vi "SetI.vi"(8 "error in (no error)":errorcluster, 10 "i":i32, 11 "reference in":refnum<class "GOOP4_Sub.lvclass">) -> (0 "error out":errorcluster, 3 "reference in":refnum<class "GOOP4_Sub.lvclass">)   [LabVIEW 2019, in "GOOP4_Sub.lvclass"]
uses:
  GOOP4_Sub.lvclass
  C:/Users/Tiba/Desktop/GOOP4_CreateObjects_Open_GDS/GOOP4_Base_class/GOOP4_Base.lvclass
  GOOP4_Base_class/GOOP4_Base.lvclass
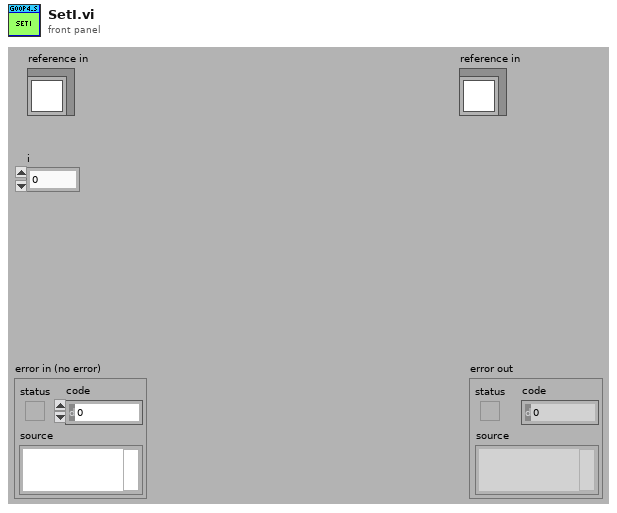
[diagram p1: front panel]
types:
  T1 = typedef "GOOP4_Base.lvclass/ObjectAttributes.ctl" = cluster{"i":i32}
  T2 = typedef "GOOP4_Sub.lvclass/ObjectAttributes.ctl" = cluster{"Str":string, "Boolean":bool}
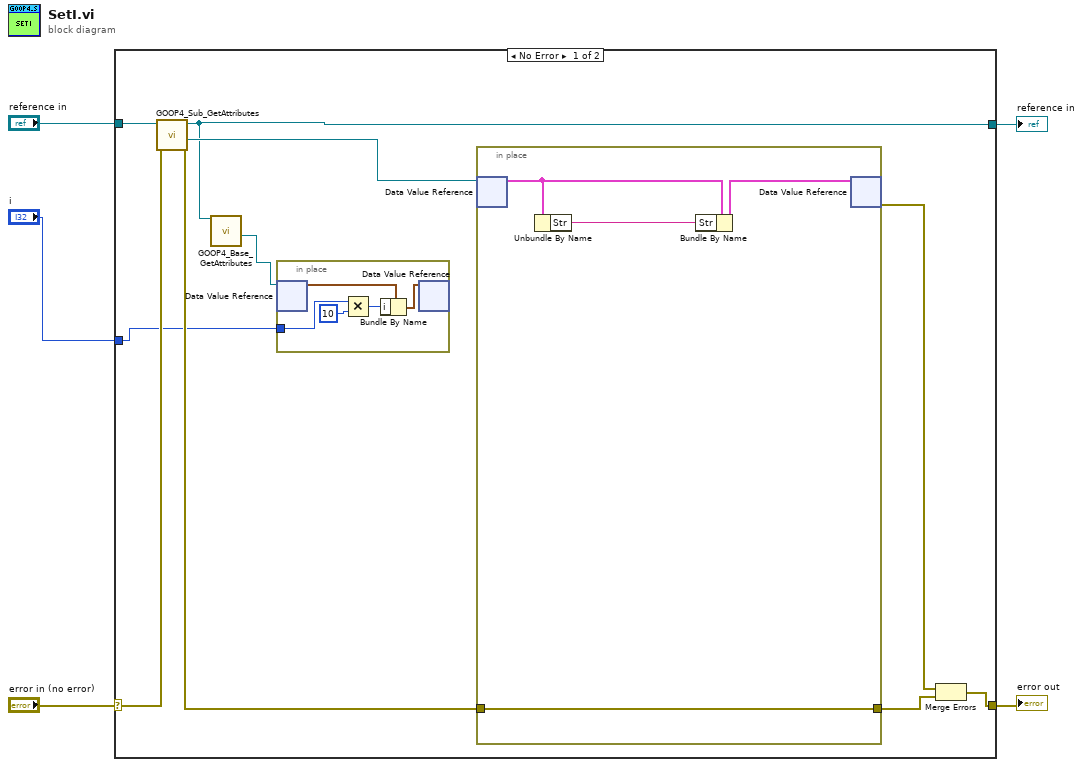
[diagram p0: block diagram]
diagram:
  n1 = case shown="No Error" "error in (no error)" {
    selector: "error in (no error)" -> [w14 w26]
    tunnel: [w12 w26] -> w4
    tunnel: [w7 w25] -> w2
    tunnel: "reference in" -> [w15 w25]
    tunnel: "i" -> [w8 _]
    frame No Error {
      n2 = call "GOOP4_Sub_GetAttributes.vi"("error in (no error)"=w14, "reference in"=w15) -> ("error out"=w10:errorcluster, "DataRef"=w11:refnum<data-value>, "reference out"=w7:refnum<class "GOOP4_Sub.lvclass">)  [unwired: 6 in, 1 out]
      n3 = call "GOOP4_Base_GetAttributes.vi"("reference in"=w7) -> ("DataRef"=w6:refnum<data-value>)  [unwired: 7 in, 3 out]
      n4 = in-place {
        in-place-border: w8 -> [w19]
        n5 = in-place-dvr #1(w6) -> (w20:T1)  [unwired: 1 out]
        n6 = Multiply(x=w19, y=10) -> (x*y=w17:i32)
        n7 = Bundle By Name(cluster=w20, "i"=w17) -> (w16:T1)
        n8 = in-place-dvr #1(w16) -> ()  [unwired: 2 out]
      }
      n9 = in-place {
        in-place-border: w10 -> [w23]
        in-place-border: [w23] -> w9
        n10 = in-place-dvr #2(w11) -> (w22:T2)  [unwired: 1 out]
        n11 = Unbundle By Name(w22) -> ("Str"=w21:string)
        n12 = Bundle By Name(cluster=w22, "Str"=w21) -> (w24:T2)
        n13 = in-place-dvr #2(w24) -> (w13:errorcluster)  [unwired: 1 out]
      }
      n14 = Merge Errors(w13, w9) -> (w12:errorcluster)
    }
    frame Error {
    }
  }
  "error out" <- w4
  "reference in" <- w2
